vi "Get number of images in a Tiff stack file.vi"(8 "error in":errorcluster, 11 "file path (use dialog)":path) -> (0 "error out":errorcluster, 2 "# of images in stack":i32, 3 "path (dup)":path)   [LabVIEW 2015, in "Tiff reader.lvlib"]
doc: "Finds out how many images are in the TIFF file stack."
uses:
  Tiff reader.lvlib
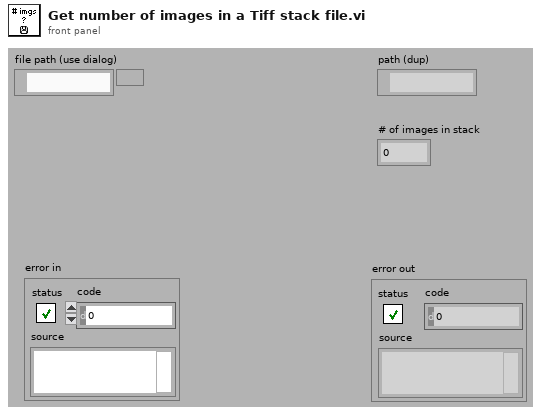
[diagram p1: front panel]
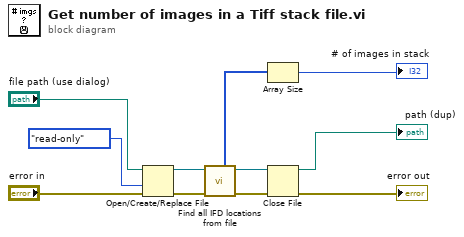
[diagram p0: block diagram]
diagram:
  n1 = Open/Create/Replace File(file path (use dialog)="file path (use dialog)", error in="error in", access (0:read/write)=enum16{"read/write", "read-only", "write-only"}."read-only") -> (refnum out=w11:refnum<file>, error out=w10:errorcluster)  [unwired: 4 out]
  n2 = call "Find all IFD locations from file.vi"("error in"=w10, "File"=w11) -> ("error out"=w8:errorcluster, "File"=w9:refnum<file>, "# of tags in each IFD"=w7:u16[])  [unwired: 7 out]
  n3 = Array Size(array=w7) -> (size(s)=→"# of images in stack":i32)
  n4 = Close File(refnum=w9, error in=w8) -> (path=→"path (dup)":path, error out=→"error out":errorcluster)
